vi "read4Byte Tx Rx.vi"(7 "address":u16, 9 "id":u8, 10 "protocol_version":i32, 11 "port_num":i32) -> (3 "function return":u32)   [LabVIEW 2016, in "dxl_x86_c.lvlib"]
doc: "WINDECLSPEC uint32_t read4ByteTxRx (int port_num, int protocol_version, uint8_t id, uint16_t address);"
uses:
  dxl_x86_c.lvlib
  dxl_x86_c.dll
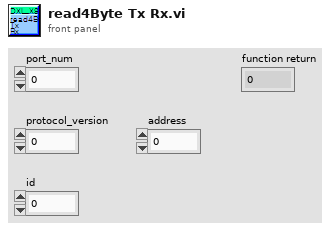
[diagram p1: front panel]
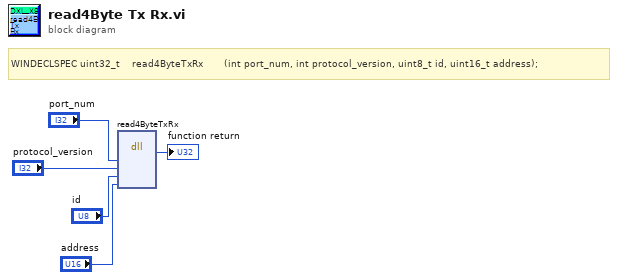
[diagram p0: block diagram]
diagram:
  # "WINDECLSPEC uint32_t    read4ByteTxRx       (int port_num, int protocol_version, uint8_t id, uint16_t address);"
  n1 = dll-call lib="C:/Users/Platform/Desktop/GITHUB/DynamixelSDK/labview/dxl_x86_c.lvlib/dxl_x86_c.*" fn="read4ByteTxRx"("port_num"="port_num", "protocol_version"="protocol_version", "id"="id", "address"="address") -> (→"function return":u32)  [unwired: 7 in, 2 out]
